vi "TCP Client.vi"() -> ()   [LabVIEW 2021]
panel:
  out "value 2":cluster{i32}
  out "value":cluster{i32}
  out "data out":string
  in  "remote port or service name":u16
  in  "address":string
  in  "Stop":bool
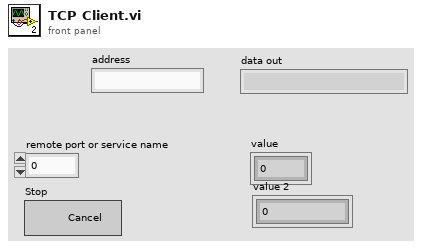
[diagram p1: front panel]
types:
  T1 = enum16{"big-endian, network order", "native, host order", "little-endian"}
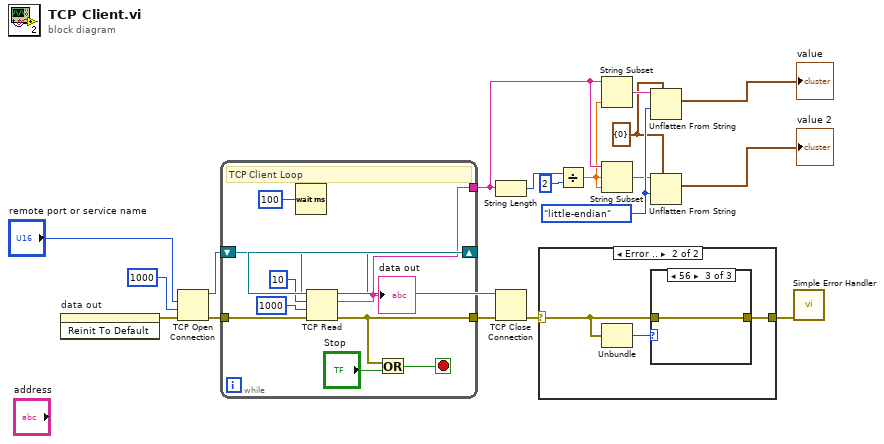
[diagram p0: block diagram]
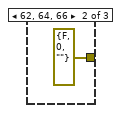
[diagram p4: hidden frame]
diagram:
  w2 = cluster{i32} {0} ("type")
  w5 = T1."little-endian" ("byte order (0:big-endian, network order)")
  n1 = invoke on="data out" class="Str" method="Reinit To Default"() -> (error out=w12:errorcluster)  [unwired: 3 in, 2 out]
  n2 = TCP Open Connection(remote port or service name="remote port or service name", timeout ms (60000)=1000, error in (no error)=w12) -> (connection ID=w11:refnum<k5>, error out=w19:errorcluster)  [unwired: 2 in]
  n3 = while {
    tunnel: w19 -> [w24]
    tunnel: [w25] -> w17
    shift-right: [w26] -> w14
    shift-left: w11 -> [w21]
    tunnel: [w20] -> w10
    stop <- w29 stop-if-true
    # "TCP Client Loop"
    n4 = Wait (ms)(milliseconds to wait=u32 100) -> ()  [unwired: 1 out]
    n5 = TCP Read(connection ID=w21, bytes to read=10, error in (no error)=w24, 9:1000 ("timeout ms (25000)")) -> (connection ID out=w26:refnum<k5>, data out=w20:string, error out=w25:errorcluster)  [unwired: 1 in]
    "data out" <- w20
    n6 = Or(x=w25, y="Stop") -> (x .or. y?=w29:bool)
  }
  n7 = String Length(string=w10) -> (length=w9:i32)
  n8 = TCP Close Connection(connection ID=w14, error in (no error)=w17) -> (error out=w16:errorcluster)  [unwired: 1 in, 1 out]
  n9 = case shown="Error .." w16 {
    selector: w16 -> [w30 w32]
    tunnel: [w30 w31] -> w15
    frame No Error {
    }
    frame Error {
      n10 = Unbundle(w32) -> ("code"=w33:i32)  [unwired: 2 out]
      n11 = case shown="56" w33 {
        tunnel: [w34 errorcluster {"status"=FALSE, "code"=0, "source"=""} ("error IO") w36] -> w31
        tunnel: w32 -> [w34 _ w36]
        frame 0, Default {
        }
        frame 62, 64, 66 {
        }
        frame 56 {
        }
      }
    }
  }
  n12 = Divide(x=w9, y=2) -> (x/y=w7:dbl)
  n13 = String Subset(string=w10, length (rest)=w7) -> (substring=w6:string)  [unwired: 1 in]
  n14 = String Subset(string=w10, offset (0)=w7, length (rest)=w7) -> (substring=w1:string)
  n15 = Unflatten From String(type=w2, binary string=w6, byte order (0:big-endian, network order)=w5) -> (value=→"value":cluster{i32})  [unwired: 2 in, 2 out]
  n16 = Unflatten From String(type=w2, binary string=w1, byte order (0:big-endian, network order)=w5) -> (value=→"value 2":cluster{i32})  [unwired: 2 in, 2 out]
  n17 = call <vilib>:"Simple Error Handler.vi"("error in (no error)"=w15) -> ()  [unwired: 4 in, 5 out]
